vi "del1tdms.vi"(4 "error in (no error)":errorcluster, 6 "names":string[](array[string]), 7 "sent time file path":path) -> (0 "error out":errorcluster)   [LabVIEW 2010]
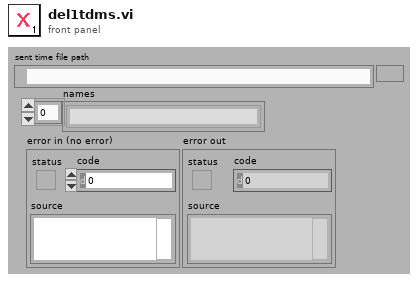
[diagram p1: front panel]
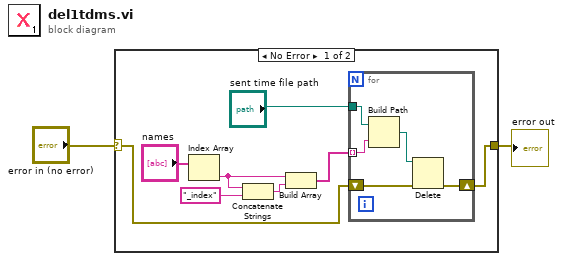
[diagram p0: block diagram]
diagram:
  n1 = case shown="No Error" "error in (no error)" {
    selector: "error in (no error)" -> [w4 w16]
    tunnel: [w3 w16] -> w1
    frame No Error {
      n2 = Index Array(array="names") -> (element=w7:string)  [unwired: 1 in]
      n3 = Concatenate Strings(w7, "_index" ("string")) -> (w8:string)
      n4 = Build Array(w7, w8) -> (w6:string[])
      n5 = for {
        tunnel: w6 -> [w15] mode=indexing
        tunnel: "sent time file path" -> [w14]
        shift-right: [w12] -> w3
        shift-left: w4 -> [w11]
        n6 = Build Path(base path=w14, name or relative path=w15) -> (appended path=w13:path)
        n7 = Delete(path (use dialog)=w13, error in=w11) -> (error out=w12:errorcluster)  [unwired: 3 in, 2 out]
      }
    }
    frame Error {
    }
  }
  "error out" <- w1
